vi "Read FoulVSS.vi"(8 "error in (no error)":errorcluster, 11 "Referee in":refnum<class "Referee.lvclass">) -> (0 "error out":errorcluster, 2 "FoulVSS":T1(ring), 3 "Referee out":refnum<class "Referee.lvclass">)   [LabVIEW 2020, in "Referee.lvclass"]
uses:
  Referee.lvclass
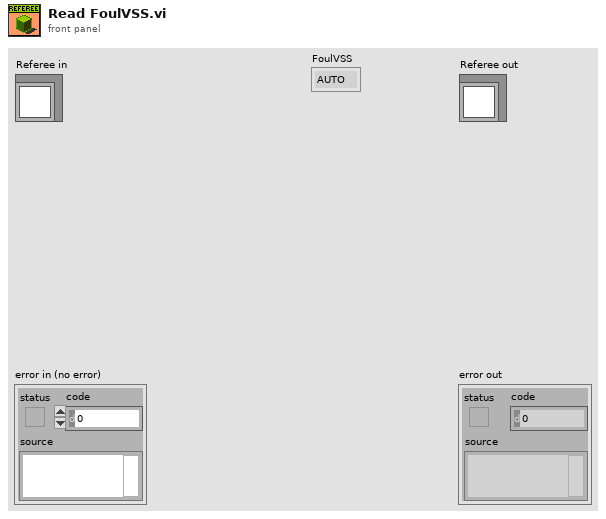
[diagram p1: front panel]
types:
  T1 = enum16{"AUTO", "GAME_ON", "STOP", "HALT", "KICKOFF", "FREE_BALL", "GOAL_KICK", "PENALTY_KICK", "FREE_KICK"}
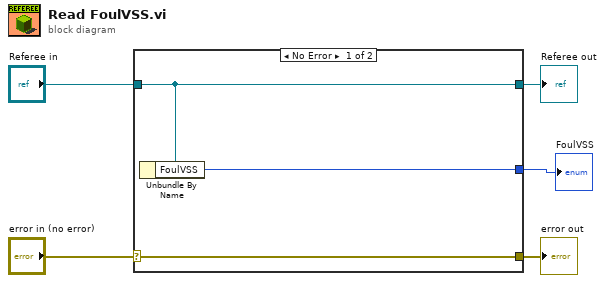
[diagram p0: block diagram]
diagram:
  n1 = case shown="No Error" "error in (no error)" {
    selector: "error in (no error)" -> [w8 w9]
    tunnel: [w8 w9] -> w4
    tunnel: [w7 w10] -> w2
    tunnel: "Referee in" -> [w7 w10]
    tunnel: [w6 _] -> w1
    frame No Error {
      n2 = Unbundle By Name(w7) -> ("FoulVSS"=w6:T1)
    }
    frame Error {
    }
  }
  "error out" <- w4
  "Referee out" <- w2
  "FoulVSS" <- w1
